vi "Obtain_arrays.vi"(0 "P Graph and Intensities and RF":cluster{"Array":dbl[], "Array":dbl[]}[](array[cluster]), 5 "Q Graph":cluster{"Array":dbl[], "Array 2":dbl[]}, 9 "Densities and De Boer":cluster{"Array":dbl[], "Array":dbl[]}[](array[cluster])) -> (1 "rho+":dbl[](array[numeric]), 2 "rho0":dbl[](array[numeric]), 3 "rho-":dbl[](array[numeric]), 4 "P":dbl[](array[numeric]), 6 "Q":dbl[](array[numeric]), 10 "RF Range 1":dbl[](array[numeric]), 11 "AFP Range":dbl[](array[numeric]), 12 "I-":dbl[](array[numeric]), 13 "De Boer":dbl[](array[numeric]), 14 "I+":dbl[](array[numeric]), 15 "RF Range 2":dbl[](array[numeric]))   [LabVIEW 2018]
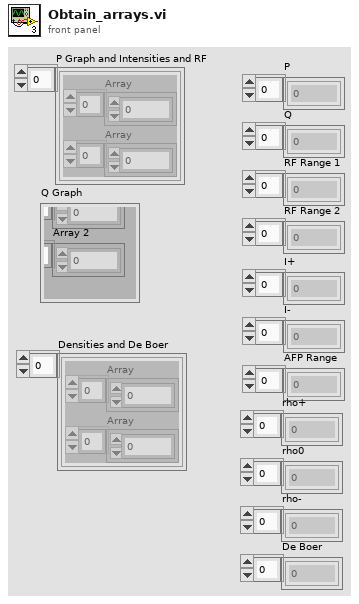
[diagram p1: front panel]
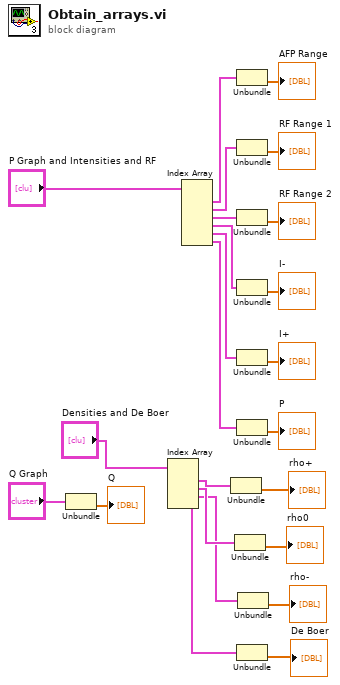
[diagram p0: block diagram]
diagram:
  n1 = Unbundle("Q Graph") -> ("Array 2"=→"Q":dbl[])  [unwired: 1 out]
  n2 = Index Array(array="Densities and De Boer") -> (element #1=w7:cluster{"Array":dbl[], "Array":dbl[]}, element #2=w6:cluster{"Array":dbl[], "Array":dbl[]}, element #3=w5:cluster{"Array":dbl[], "Array":dbl[]}, element #4=w4:cluster{"Array":dbl[], "Array":dbl[]})  [unwired: 4 in]
  n3 = Index Array(array="P Graph and Intensities and RF") -> (element #1=w22:cluster{"Array":dbl[], "Array":dbl[]}, element #2=w21:cluster{"Array":dbl[], "Array":dbl[]}, element #3=w17:cluster{"Array":dbl[], "Array":dbl[]}, element #4=w18:cluster{"Array":dbl[], "Array":dbl[]}, element #5=w19:cluster{"Array":dbl[], "Array":dbl[]}, element #6=w20:cluster{"Array":dbl[], "Array":dbl[]})  [unwired: 6 in]
  n4 = Unbundle(w7) -> ("Array"=→"rho+":dbl[])  [unwired: 1 out]
  n5 = Unbundle(w6) -> ("Array"=→"rho0":dbl[])  [unwired: 1 out]
  n6 = Unbundle(w22) -> ("Array"=→"AFP Range":dbl[])  [unwired: 1 out]
  n7 = Unbundle(w21) -> ("Array"=→"RF Range 1":dbl[])  [unwired: 1 out]
  n8 = Unbundle(w17) -> ("Array"=→"RF Range 2":dbl[])  [unwired: 1 out]
  n9 = Unbundle(w18) -> ("Array"=→"I-":dbl[])  [unwired: 1 out]
  n10 = Unbundle(w19) -> ("Array"=→"I+":dbl[])  [unwired: 1 out]
  n11 = Unbundle(w20) -> ("Array"=→"P":dbl[])  [unwired: 1 out]
  n12 = Unbundle(w4) -> ("Array"=→"De Boer":dbl[])  [unwired: 1 out]
  n13 = Unbundle(w5) -> ("Array"=→"rho-":dbl[])  [unwired: 1 out]
